vi "Merge Config Files.vi"(6 "Version Prompt (F)":bool, 7 "Server is Source (T)":bool=TRUE, 8 "Error IN":errorcluster, 10 "Dest Path":path, 11 "Source Path":path) -> (0 "Error OUT":errorcluster)   [LabVIEW 2023]
uses:
  Type Defs and Controls/Sensor Config.ctl
  Type Defs and Controls/DAQ Settings.ctl
  Type Defs and Controls/Trigger Stop Method.ctl
  Type Defs and Controls/Log File Type.ctl
  Type Defs and Controls/Channel Config.ctl
  Type Defs and Controls/Header.ctl
  Type Defs and Controls/Graph Settings Type Def.ctl
  Type Defs and Controls/Test Limits.ctl
  Type Defs and Controls/All Part Info.ctl
  Type Defs and Controls/Part Info.ctl
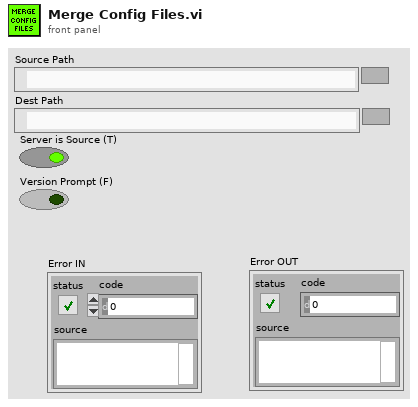
[diagram p1: front panel]
types:
  T1 = enum16{"Left Button", "Center Button", "Right Button", "Window Close"}
  T2 = typedef "Sensor Config.ctl" = cluster{"DAQ Settings":T3, "Channels":T6[], "Header":T7, "Graph Settings":T8, "Test Limits":T9[], "All Type Info":T10, "Save Mode":enum16{"Single File", "Segmented Files", "New File at Midnight"}, "Data Base Path":path}
  T3 = typedef "DAQ Settings.ctl" = cluster{"Trigger Type":enum16{"Manual", "Timed", "Analog Rising", "Analog Falling"}, "Trigger Samples":i32, "Pretrigger Samples":i32, "Trigger Interval":dbl, "Time Units":bool, "Auto Save":bool, "Sample Rate":dbl, "Select Analog":bool, "Trigger Value":dbl, "Trigger Stop Method":T4, "Rate Sec/Min":bool, "Save Mode":enum16{"Single File", "Segmented Files", "New File at Midnight"}, "File Size Limit":dbl, "Log File Type":T5, "Trigger Data Index":u32, "Log Rate":dbl, "Rate Sec/Min (Log)":bool, "Sample Rate (S/s)":dbl, "Log Rate (S/s)":dbl}
  T4 = typedef "Trigger Stop Method.ctl" = enum16{"Use Samples Value to Stop Trigger", "Use Threshold to Stop Trigger"}
  T5 = typedef "Log File Type.ctl" = enum16{"Basic", "RTS"}
  T6 = typedef "Channel Config.ctl" = cluster{"Channel":string, "Type":string, "Acquire":bool, "Name":string, "Sensor":string, "Data Index":u32}
  T7 = typedef "Header.ctl" = cluster{"CA Number":string, "Test Name":string, "Serial Number":string, "Technician":string}
  T8 = typedef "Graph Settings Type Def.ctl" = cluster{"Graph Labels":string[], u8[], i16[], u32[], u8[], u8[], u8[], u32[], u8[], u8[], u8[], dbl[], dbl[], "Graph Toggles":bool[], "Axis Toggles":bool[], "Graph Range":enum16{"1", "2", "3", "4", "5", "10", "15", "30", "60"}}
  T9 = typedef "Test Limits.ctl" = cluster{"Channel Acquired?":bool, "RMS?":bool, "Pk-Pk":bool, "Frequency":bool, "EU High Limit 1":dbl, "EU Low Limit 1":dbl, "EU High Limit 2":dbl, "EU Low Limit 2":dbl, "RMS High Limit":dbl, "RMS Low Limit":dbl, "Pk-Pk High Limit ":dbl, "Pk-Pk Low Limit":dbl, "Frequency High Limit":dbl, "Frequency Low Limit":dbl}
  T10 = typedef "All Part Info.ctl" = cluster{"Type Name":string, "Type Signal Names":string[], "# Signals":i32, "# Parts":i32, "Part Info":T11[]}[]
  T11 = typedef "Part Info.ctl" = cluster{"Part Number":string, "Channel Indexes":u16[], "Enabled?":bool}
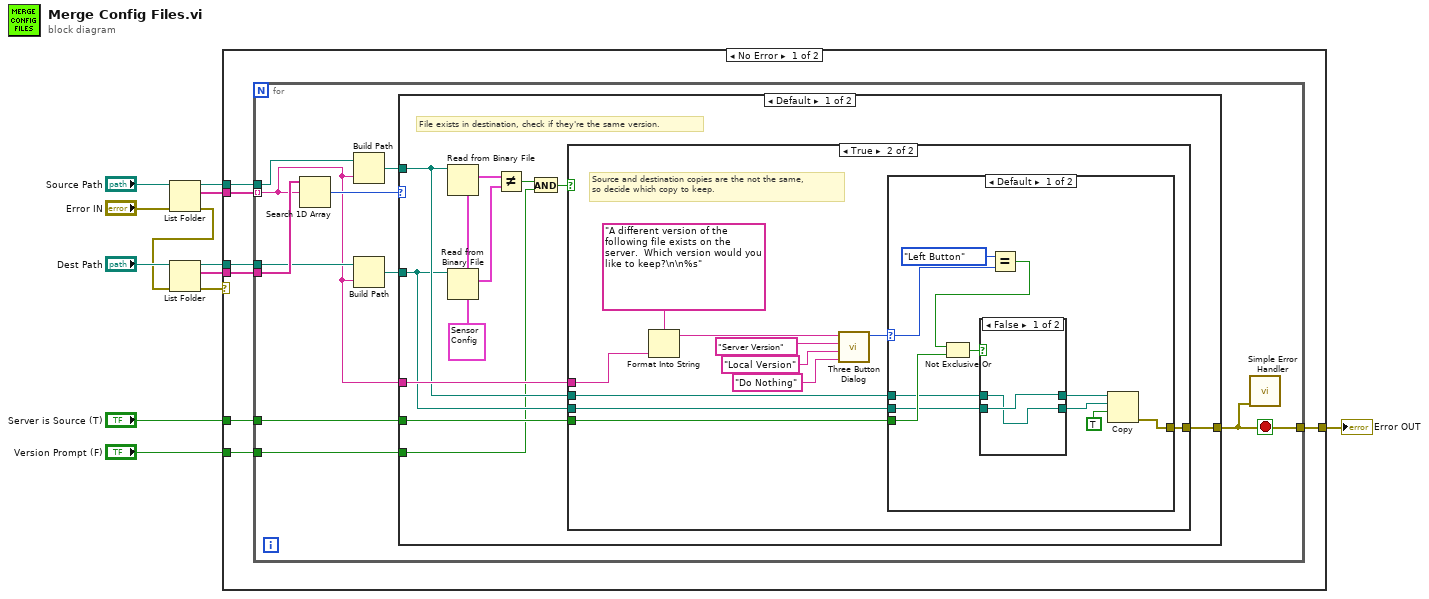
[diagram p0: block diagram]
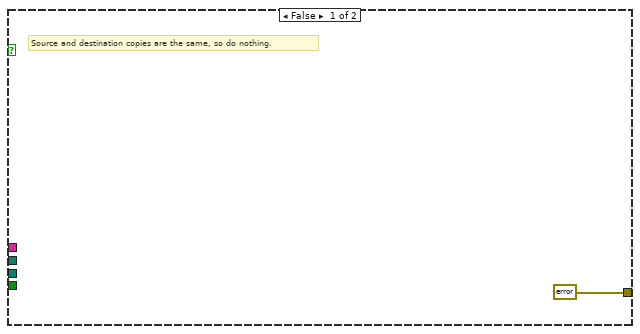
[diagram p2: hidden frame]
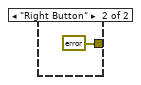
[diagram p4: hidden frame]
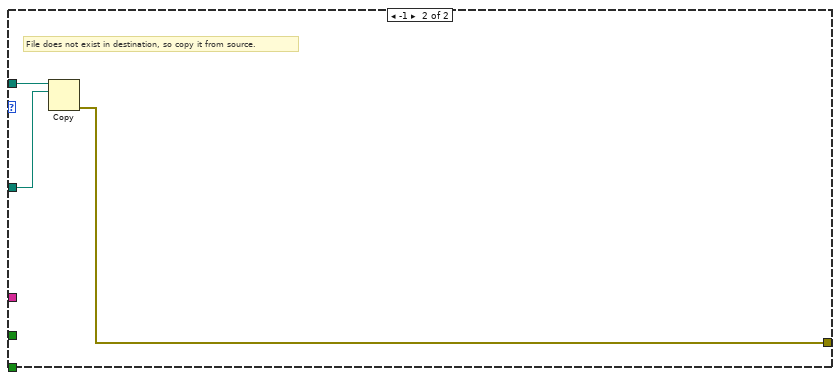
[diagram p5: hidden frame]
diagram:
  n1 = List Folder(path="Source Path", error in="Error IN") -> (path out=w8:path, filenames=w10:string[], error out=w2:errorcluster)  [unwired: 2 in, 1 out]
  n2 = List Folder(path="Dest Path", error in=w2) -> (path out=w7:path, filenames=w9:string[], error out=w1:errorcluster)  [unwired: 2 in, 1 out]
  n3 = case shown="No Error" w1 {
    selector: w1 -> [_ w72]
    tunnel: w10 -> [w19 _]
    tunnel: w9 -> [w18 _]
    tunnel: w8 -> [w17 _]
    tunnel: w7 -> [w16 _]
    tunnel: "Server is Source (T)" -> [w15 _]
    tunnel: [w14 w72] -> w5
    tunnel: "Version Prompt (F)" -> [w13 _]
    frame No Error {
      n4 = for {
        tunnel: w19 -> [w23] mode=indexing
        tunnel: w18 -> [w29]
        tunnel: w17 -> [w26]
        tunnel: w16 -> [w27]
        tunnel: w15 -> [w22]
        tunnel: [w21] -> w14
        tunnel: w13 -> [w20]
        stop <- w21 stop-if-true
        n5 = Search 1D Array(1D array=w29, element=w23) -> (index of element=w28:i32)  [unwired: 1 in]
        n6 = Build Path(base path=w26, name or relative path=w23) -> (appended path=w24:path)
        n7 = Build Path(base path=w27, name or relative path=w23) -> (appended path=w25:path)
        n8 = case shown="Default" w28 {
          tunnel: [w39 w71] -> w21
          tunnel: w25 -> [w35 w70]
          tunnel: w24 -> [w36 w69]
          tunnel: w23 -> [w38 _]
          tunnel: w22 -> [w37 _]
          tunnel: w20 -> [w33 _]
          frame Default {
            w40 = T2 {"DAQ Settings"={"Trigger Type"=enum."Manual", "Trigger Samples"=0, "Pretrigger Samples"=0, "Trigger Interval"=0.0, "Time Units"=FALSE, "Auto Save"=FALSE, "Sample Rate"=0.0, "Select Analog"=FALSE, "Trigger Value"=0.0, "Trigger Stop Method"=enum."Use Samples Value to Stop Trigger", "Rate Sec/Min"=FALSE, "Save Mode"=enum."Single File", "File Size Limit"=0.0, "Log File Type"=enum."Basic", "Trigger Data Index"=0, "Log Rate"=7.0, "Rate Sec/Min (Log)"=FALSE, "Sample Rate (S/s)"=0.0, "Log Rate (S/s)"=0.0}, "Channels"=[], "Header"={"CA Number"="", "Test Name"="", "Serial Number"="", "Technician"=""}, "Graph Settings"={"Graph Labels"=[], [], [], [], [], [], [], [], [], [], [], [], [], "Graph Toggles"=[], "Axis Toggles"=[], "Graph Range"=enum."1"}, "Test Limits"=[], "All Type Info"=[], "Save Mode"=enum."Single File", "Data Base Path"=path ""} ("Config")
            # "File exists in destination, check if they're the same version."
            n9 = Read from Binary File(5:w40, 11:w36) -> (2:w31:T2)  [unwired: 4 in, 3 out]
            n10 = Read from Binary File(5:w40, 11:w35) -> (2:w30:T2)  [unwired: 4 in, 3 out]
            n11 = Not Equal?(x=w31, y=w30) -> (x != y?=w34:bool)
            n12 = And(x=w34, y=w33) -> (x .and. y?=w32:bool)
            n13 = case shown="True" w32 {
              tunnel: [errorcluster {"status"=FALSE, "code"=0, "source"=""} ("error out") w47] -> w39
              tunnel: w38 -> [_ w52]
              tunnel: w37 -> [_ w50]
              tunnel: w36 -> [_ w49]
              tunnel: w35 -> [_ w48]
              frame False {
                # "Source and destination copies are the same, so do nothing."
              }
              frame True {
                # "Source and destination copies are the not the same,\nso decide which copy to keep."
                n14 = Format Into String(format string="A different version of the following file exists on the server.  Which version would you like to keep?\n\n%s" ("message"), w52) -> (resulting string=w51:string)  [unwired: 2 in, 1 out]
                n15 = call <vilib>:"Three Button Dialog.vi"("Right Button Text (\"Cancel\")"="Do Nothing" ("T button name (\"OK\")"), "Center Button Text (\"No\")"="Local Version" ("T button name (\"OK\")"), "Left Button Text (\"Yes\")"="Server Version" ("T button name (\"OK\")"), "message"=w51) -> ("Which Button?"=w42:T1)  [unwired: 7 in]
                n16 = case shown="Default" w42 {
                  selector: w42 -> [w55 _]
                  tunnel: w50 -> [w63 _]
                  tunnel: w49 -> [w61 _]
                  tunnel: w48 -> [w60 _]
                  tunnel: [w57 errorcluster {"status"=FALSE, "code"=0, "source"=""} ("error out")] -> w47
                  frame Default {
                    n17 = Equal?(x=T1."Left Button", y=w55) -> (x = y?=w53:bool)
                    n18 = Not Exclusive Or(1:w63, 2:w53) -> (0:w62:bool)
                    n19 = case shown="False" w62 {
                      tunnel: w61 -> [w64 w67]
                      tunnel: w60 -> [w65 w66]
                      tunnel: [w65 w67] -> w59
                      tunnel: [w64 w66] -> w58
                      frame False {
                      }
                      frame True {
                      }
                    }
                    n20 = Copy(9:TRUE ("overwrite (F)"), 10:w58, 11:w59) -> (0:w57:errorcluster)  [unwired: 2 in, 2 out]
                  }
                  frame "Right Button" {
                  }
                }
              }
            }
          }
          frame -1 {
            # "File does not exist in destination, so copy it from source."
            n21 = Copy(10:w70, 11:w69) -> (0:w71:errorcluster)  [unwired: 3 in, 2 out]
          }
        }
        n22 = call <vilib>:"Simple Error Handler.vi"("error in (no error)"=w21) -> ()  [unwired: 4 in, 5 out]
      }
    }
    frame Error {
    }
  }
  "Error OUT" <- w5
